vi "Pixie4Bootuser.vi"(1 "Select PXI chassis type":T1=enum."18-slot chassis", 2 "Offline analysis ?":bool, 3 "Module #":u16[](array[numeric])=[8, 4] caption="PXI Slot #" min=2 max=18 step=1, 4 "Total number of Pixie-4 modules":u16=1 min=1 max=17 step=1, 5 "DSP memory variable file (.lst file in folder \"DSP\")":path=path "C:/Program Files (x86)/National Instruments/LabVIEW 2016/user.lib/DSP/PXIcode.lst", 6 "DSP I/O variable file (.var file in folder \"DSP\")":path=path "C:/Program Files (x86)/National Instruments/LabVIEW 2016/user.lib/DSP/PXIcode.var", 7 "DSP parameters file (.set file in folder \"Configuration\")":path=path "D:/dsp files/I129/final.set", 8 "DSP executable code file (.bin file in folder DSP\")":path=path "C:/Program Files (x86)/National Instruments/LabVIEW 2016/user.lib/DSP/PXIcode.bin", 9 "Signal proceesing FPGA file (.bin file in folder \"Firmware\")":path=path "C:/Program Files (x86)/National Instruments/LabVIEW 2016/user.lib/Firmware/pixie.bin", 10 "Communication FPGA file for REVC (.bin file in folder \"Firmware\")":path=path "C:/Program Files (x86)/National Instruments/LabVIEW 2016/user.lib/Firmware/syspixie_revC.bin", 11 "Communication FPGA file for REVB (.bin file in folder \"Firmware\")":path=path "C:/Program Files (x86)/National Instruments/LabVIEW 2016/user.lib/Firmware/FippiP500.bin") -> (0 "Return value for booting":i32)   [LabVIEW 2016]
uses:
  controls/pixie crates.ctl
  Drivers/Pixie4DLL.dll
panel:
  # "0  - boot successful\n-1  - unable to scan the PXI crate slots\n-2  - unable to read communication FPGA configuration (Rev. B)\n-3  - unable to read communication FPGA configuration (Rev. C)\n-4  - unable to read signal processing FPGA configuration\n-5  - unable to read DSP executable code\n-6  - unable to read DSP parameter values\n-7  - unable to initialize DSP parameter names\n-8  - failed to boot all modules present in the system\n-9  - failed to initialize NUMBER_MODULES\n-10- failed to initialize OFFLINE_ANALYSIS\n-11- failed to initialize MAX_NUMBER_MODULES\n-12- failed to initialize SLOT_WAVE"
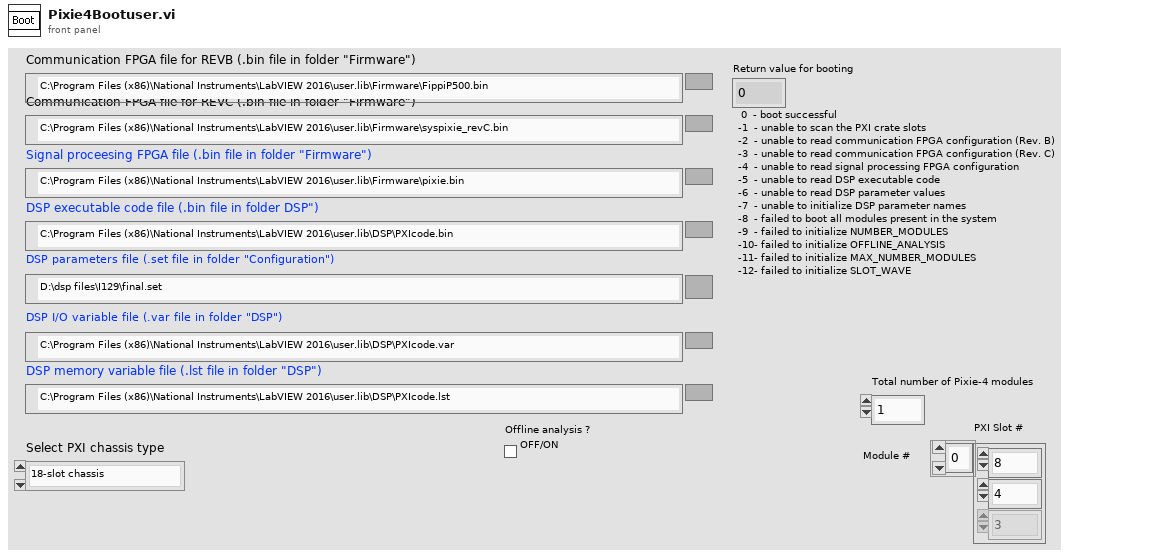
[diagram p1: front panel]
types:
  T1 = typedef "pixie crates.ctl" = enum16{"4 or 8-slot chassis", "14-slot chassis", "18-slot chassis"}
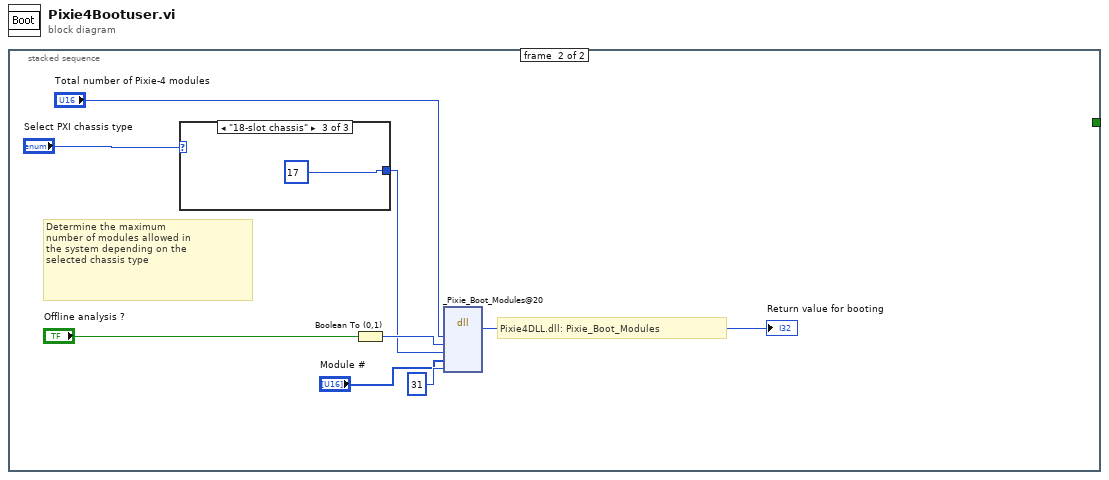
[diagram p0: block diagram]
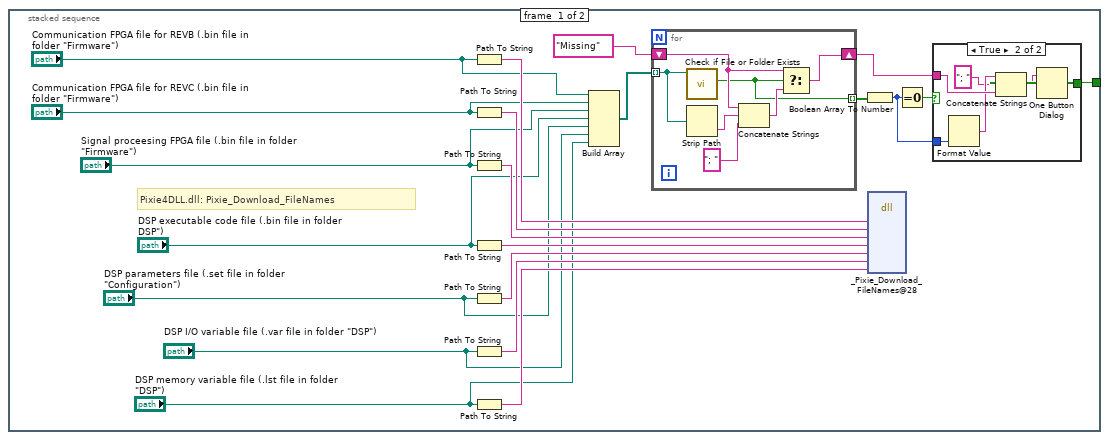
[diagram p2: hidden frame]
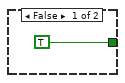
[diagram p3: hidden frame]
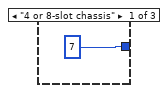
[diagram p4: hidden frame]
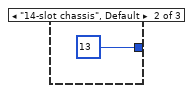
[diagram p5: hidden frame]
diagram:
  n1 = stacked-sequence {
    tunnel: [w4 _] -> _
    frame #0 {
      # "Pixie4DLL.dll: Pixie_Download_FileNames"
      n2 = Path To String(path="Communication FPGA file for REVB (.bin file in folder \"Firmware\")") -> (string=w15:string)
      n3 = Path To String(path="Communication FPGA file for REVC (.bin file in folder \"Firmware\")") -> (string=w16:string)
      n4 = Path To String(path="Signal proceesing FPGA file (.bin file in folder \"Firmware\")") -> (string=w17:string)
      n5 = Path To String(path="DSP executable code file (.bin file in folder DSP\")") -> (string=w18:string)
      n6 = Path To String(path="DSP parameters file (.set file in folder \"Configuration\")") -> (string=w19:string)
      n7 = Path To String(path="DSP I/O variable file (.var file in folder \"DSP\")") -> (string=w20:string)
      n8 = Path To String(path="DSP memory variable file (.lst file in folder \"DSP\")") -> (string=w21:string)
      n9 = Build Array("Communication FPGA file for REVB (.bin file in folder \"Firmware\")", "Communication FPGA file for REVC (.bin file in folder \"Firmware\")", "Signal proceesing FPGA file (.bin file in folder \"Firmware\")", "DSP executable code file (.bin file in folder DSP\")", "DSP parameters file (.set file in folder \"Configuration\")", "DSP I/O variable file (.var file in folder \"DSP\")", "DSP memory variable file (.lst file in folder \"DSP\")") -> (w7:path[])
      n10 = for {
        tunnel: w7 -> [w35] mode=indexing
        shift-right: [w34] -> w5
        shift-left: "Missing" -> [w32]
        tunnel: [w29] -> w3 mode=indexing
        n11 = call <vilib>:"Check if File or Folder Exists.vi"("path"=w35) -> ("file or folder exists?"=w29:bool)  [unwired: 8 in, 2 out]
        n12 = Strip Path(path=w35) -> (name=w31:string)  [unwired: 1 out]
        n13 = Concatenate Strings(w32, w31, "; " ("string")) -> (w33:string)
        n14 = Select(t=w32, s=w29, f=w33) -> (s? t:f=w34:string)
      }
      n15 = Boolean Array To Number(Boolean array=w3) -> (number=w1:u32)
      n16 = dll-call lib="D:/Users/wymanm/Desktop/DAQuiri - 2017a/lois/Drivers/Pixie4DLL.dll" fn="_Pixie_Download_FileNames@28" label="Call Library Function"("ComFPGAFileNameRevB"=w15, "ComFPGAFileNameRevC"=w16, "SPFPGAFileName"=w17, "DSPCodeFileName"=w18, "DSPParFileName"=w19, "DSPVarFileName"=w20, "DSPLstFileName"=w21) -> ()  [unwired: 11 in, 2 out]
      n17 = Equal To 0?(x=w1) -> (x = 0?=w2:bool)
      n18 = case shown="True" w2 {
        tunnel: w5 -> [_ w27]
        tunnel: [TRUE ("true") w28] -> w4
        tunnel: w1 -> [_ w25]
        frame False {
        }
        frame True {
          n19 = Format Value(value (0)=w25) -> (output string=w24:string)  [unwired: 2 in]
          n20 = Concatenate Strings(w24, "; ", w27) -> (w26:string)
          n21 = One Button Dialog(message=w26) -> (true=w28:bool)  [unwired: 1 in]
        }
      }
    }
    frame #1 {
      # "Pixie4DLL.dll: Pixie_Boot_Modules"
      # "Determine the maximum\nnumber of modules allowed in\nthe system depending on the\nselected chassis type"
      n22 = case shown="\"18-slot chassis\"" "Select PXI chassis type" {
        tunnel: [u16 7 u16 13 ("MaxNumberOfModules") u16 17] -> w36
        frame "4 or 8-slot chassis" {
        }
        frame "14-slot chassis", Default {
        }
        frame "18-slot chassis" {
        }
      }
      n23 = Boolean To (0,1)(Boolean="Offline analysis ?") -> (0, 1=w40:i16)
      n24 = dll-call lib="D:/Users/wymanm/Desktop/DAQuiri - 2017a/lois/Drivers/Pixie4DLL.dll" fn="_Pixie_Boot_Modules@20" label="Call Library Function"("TotalNumberModules"="Total number of Pixie-4 modules", "OfflineAnalysis"=w40, "MaxNumberOfModules"=w36, "PXISlotMap"="Module #", "BootPattern"=u16 31) -> ("return type"=→"Return value for booting":i32)  [unwired: 8 in, 2 out]
    }
  }
